vi "HFRR ADV v07 new software.vi"() -> ()   [LabVIEW 2025] (continued)
                    n2724 = Concatenate Strings(w3585, ".xls" ("string")) -> (w3583:string)
                  }
                  frame "csv" {
                    n2725 = Concatenate Strings(w3587, ".csv" ("string")) -> (w3588:string)
                  }
                  frame "txt" {
                    n2726 = Concatenate Strings(w3589, ".txt" ("string")) -> (w3590:string)
                  }
                }
                n2727 = local read "Test Date"() -> (w3581:string)
                n2728 = local read "String 45"() -> (w3495:string)
                n2729 = local read "String 31"() -> (w3580:string)
                n2730 = local read "String 32"() -> (w3579:string)
                n2731 = local read "TITTLE"() -> (w3503:string)
                n2732 = Number To Fractional String(number=w3550, width (-)=i16 6, precision (6)=i16 2) -> (F-format string=w3549:string)  [unwired: 1 in]
                n2733 = Number To Fractional String(number=w3564, width (-)=i16 6, precision (6)=i16 2) -> (F-format string=w3570:string)  [unwired: 1 in]
                n2734 = Number To Fractional String(number=w3565, width (-)=i16 6, precision (6)=i16 2) -> (F-format string=w3563:string)  [unwired: 1 in]
                n2735 = Number To Fractional String(number=w3569, width (-)=i16 6, precision (6)=i16 2) -> (F-format string=w3568:string)  [unwired: 1 in]
                n2736 = Number To Fractional String(number=w3561, width (-)=i16 6, precision (6)=i16 2) -> (F-format string=w3559:string)  [unwired: 1 in]
                n2737 = Number To Fractional String(number=w3562, width (-)=i16 6, precision (6)=i16 2) -> (F-format string=w3560:string)  [unwired: 1 in]
                n2738 = Number To Fractional String(number=w3573, width (-)=i16 6, precision (6)=i16 2) -> (F-format string=w3574:string)  [unwired: 1 in]
                n2739 = Number To Fractional String(number=w3577, precision (6)=i16 2) -> (F-format string=w3578:string)  [unwired: 2 in]
                n2740 = local read "s.NO"() -> (w3497:string)
                n2741 = Concatenate Strings("=" ("string"), w3503) -> (w3502:string)
                n2742 = Concatenate Strings("S.No," ("string"), "                                       Parameters" ("string")) -> (w3508:string)
                n2743 = Concatenate Strings(w3575, w3534, w3549, w3575, w3531, w3570, w3575, w3530, w3563, w3575, w3526, w3568, w3575, w3524, w3559, w3575, w3521, w3560, w3575, w3518, w3574, w3575, w3515, w3578) -> (w3537:string)
                n2744 = Concatenate Strings(w3507, "," ("string"), w3495, w3497, w3496, w3579, w3582, w3496, w3580, w3581, w3507) -> (w3505:string)
                n2745 = local read "Tested by"() -> (w3511:string)
                n2746 = local read "String 33"() -> (w3512:string)
                n2747 = Concatenate Strings("," ("string"), "                                                                             " ("string")) -> (w3500:string)
                n2748 = Concatenate Strings(w3502, w3498, w3505, w3498, w3508, w3537, w3498, w3500, w3512, w3511) -> (→"export":string)
                n2749 = String To Path(string=w3539) -> (path=w3546:path)
                n2750 = local read "export"() -> (w3541:string)
                n2751 = call <vilib>:"Write Characters To File.vi"("append to file? (new file:F)"=FALSE, "character string"=w3541, "file path (dialog if empty)"=w3546) -> ()  [unwired: 2 in, 1 out]
              }
            }
          }
          frame Enabled {
          }
        }
        n2752 = case shown="True" "OK Button 17" {
          frame False {
          }
          frame True {
            (unwired) 0  # existing file
            w3799 = "Choose a datalog file to open"  # prompt
            n2753 = local write "OK Button 17"(FALSE ("OK Button 17")) -> ()
            n2754 = local read "String"() -> (w3794:string)
            n2755 = String To Path(string=w3794) -> (path=w3795:path)
            n2756 = File Dialog(6:"*.duf" ("pattern"), 7:w3799, 11:w3795) -> (0:w3786:errorcluster, 3:w3805:path)  [unwired: 4 in, 2 out]
            n2757 = Unbundle(w3786) -> ()  [unwired: 3 out]
            n2758 = Open/Create/Replace File "Open File"(file path (use dialog)=w3805) -> (refnum out=w3797:refnum<file>)  [unwired: 5 in, 2 out]
            n2759 = Strip Path(path=w3805) -> (name=w3803:string)  [unwired: 1 out]
            n2760 = Path To String(path=w3805) -> (string=w3788:string)
            n2761 = while {
              tunnel: w3797 -> [w3809]
              i -> [w3806]
              stop <- w3807 continue-if-true
              (unwired) TRUE ("line mode (F)")
              n2762 = Read from Text File "Read File"(file (use dialog)=w3809) -> (text=w3808:string)  [unwired: 3 in, 3 out]
              n2763 = local write "Numeric 16"(w3806) -> ()
              n2764 = String Length(string=w3808) -> (length=w3811:i32)
              n2765 = Greater?(x=w3811, y=1) -> (0:w3807:bool)
            }
            n2766 = local write "String 29"(w3788) -> ()
            n2767 = Search and Replace String(input string=w3788, search string=".duf", replace string=".dgf" ("replace string (\"\")")) -> (result string=→"String Indicator 4":string)  [unwired: 5 in, 3 out]
            n2768 = Match Pattern(string=w3803, regular expression=".dwm") -> (before substring=w3787:string)  [unwired: 1 in, 3 out]
            "String Indicator" <- w3787
            n2769 = Match Pattern(string=w3788, regular expression=".dwm" ("substring (\"\")")) -> (before substring=w3789:string)  [unwired: 1 in, 3 out]
            "String Indicator 3" <- w3789
            n2770 = local write "TITTLE 2"(w3787) -> ()
            n2771 = String To Path(string=w3789) -> (path=w3796:path)
            "path" <- w3796
            n2772 = call <vilib>:"Read Characters From File.vi"("file path (dialog if empty)"=w3796, "start of read offset (chars.:0)"=60 ("start of read offset (chars.: 0)")) -> ("character string"=→"String Indicator 2":string)  [unwired: 4 in, 3 out]
          }
        }
        n2773 = call <vilib>:"Query Available Printers.vi"() -> ("system configured printers"=w3488:string[])  [unwired: 9 in, 2 out]
        "System Configured Printers 2" <- w3488
        n2774 = local read "OK Button 16"() -> (w3485:bool)
        n2775 = case shown="True" "OK Button 16" {
          frame False {
          }
          frame True {
            n2776 = stacked-sequence {
              frame #0 {
                n2777 = local read "Numeric 16"() -> (w3813:i32)
                n2778 = local write "Numeric 10"(w3813) -> ()
              }
              frame #1 {
                n2779 = local read "S.NO"() -> (→"s.NO":string)
                n2780 = local read "String 29"() -> (w3817:string)
                n2781 = String To Path(string=w3817) -> (path=w3816:path)
                n2782 = Open/Create/Replace File "Open File"(file path (use dialog)=w3816) -> (refnum out=w3818:refnum<file>)  [unwired: 5 in, 2 out]
                n2783 = for {
                  N: 16 -> [_]
                  tunnel: w3818 -> [w3825]
                  i -> [w3821]
                  (unwired) TRUE ("line mode (F)")
                  n2784 = Read from Text File "Read File"(file (use dialog)=w3825) -> (text=w3819:string)  [unwired: 3 in, 3 out]
                  n2785 = Match Pattern(string=w3819, regular expression="(") -> (after substring=w3824:string)  [unwired: 1 in, 3 out]
                  n2786 = Match Pattern(string=w3824, regular expression=")") -> (before substring=w3820:string)  [unwired: 1 in, 3 out]
                  n2787 = case shown="1" w3821 {
                    tunnel: w3820 -> [w3826 w3827 _ _ w3828 w3829 w3830 w3832 w3834 w3836 w3838 w3840 w3842 w3844 _]
                    tunnel: w3819 -> [_ _ _ _ _ _ _ _ _ _ _ _ _ _ _]
                    frame 0 {
                      "TITTLE" <- w3826
                    }
                    frame 1 {
                      "Sample ID" <- w3827
                    }
                    frame 2 {
                    }
                    frame 3 {
                    }
                    frame 4 {
                      "Test Date" <- w3828
                    }
                    frame 5 {
                      "Tested by" <- w3829
                    }
                    frame 6 {
                      n2788 = Fract/Exp String To Number(string=w3830) -> (number=→"Humidity before test 2":dbl)  [unwired: 3 in, 1 out]
                    }
                    frame 7 {
                      n2789 = Fract/Exp String To Number(string=w3832) -> (number=→"Temperature before test 2":dbl)  [unwired: 3 in, 1 out]
                    }
                    frame 8 {
                      n2790 = Fract/Exp String To Number(string=w3834) -> (number=→"Humidity after test 2":dbl)  [unwired: 3 in, 1 out]
                    }
                    frame 9 {
                      n2791 = Fract/Exp String To Number(string=w3836) -> (number=→"Temperature after test 2":dbl)  [unwired: 3 in, 1 out]
                    }
                    frame 10 {
                      n2792 = Fract/Exp String To Number(string=w3838) -> (number=→"MWSD 2":dbl)  [unwired: 3 in, 1 out]
                    }
                    frame 11 {
                      n2793 = Fract/Exp String To Number(string=w3840) -> (number=→"AVP 2":dbl)  [unwired: 3 in, 1 out]
                    }
                    frame 12 {
                      n2794 = Fract/Exp String To Number(string=w3842) -> (number=→"HCF 2":dbl)  [unwired: 3 in, 1 out]
                    }
                    frame 13 {
                      n2795 = Fract/Exp String To Number(string=w3844) -> (number=→"WS1.4 2":dbl)  [unwired: 3 in, 1 out]
                    }
                    frame 14, Default {
                    }
                  }
                }
              }
              frame #2 {
              }
            }
            n2796 = local write "OK Button 16"(FALSE ("OK Button 13")) -> ()
          }
        }
        n2797 = Index Array(array=w3488, index="Select Printer 3") -> (element=w3490:string)
        "Selected Printer" <- w3490
        n2798 = case shown="True" w3485 {
          frame False {
          }
          frame True {
            n2799 = flat-sequence {
              frame #0 {
              }
              frame #1 {
                n2800 = Wait (ms)(milliseconds to wait=u32 100) -> ()  [unwired: 1 out]
              }
              frame #2 {
                n2801 = local write "OK Button 16"(FALSE ("Print 3")) -> ()
              }
            }
          }
        }
        n2802 = case shown="True" "Print" {
          tunnel: w3490 -> [_ w3782]
          frame False {
          }
          frame True {
            (unwired) i16 6 ("width (-)")
            (unwired) "TESTED BY : "
            (unwired) "TESTED DATE :"
            (unwired) "SAMPLE ID : "
            (unwired) "SAMPLE DESIGN : "
            w3740 = "\r"
            w3757 = "\r"
            # "add image"
            n2803 = local read "Sample ID"() -> (w3730:string)
            n2804 = local read "Tested by"() -> (w3733:string)
            n2805 = local read "String 34"() -> (w3720:string)
            n2806 = local read "String 45"() -> (w3700:string)
            n2807 = local read "String 35"() -> (w3715:string)
            n2808 = local read "String 37"() -> (w3713:string)
            n2809 = local read "String 32"() -> (w3735:string)
            n2810 = local read "String 36"() -> (w3710:string)
            n2811 = local read "String 31"() -> (w3734:string)
            n2812 = local read "Test Date"() -> (w3731:string)
            n2813 = local read "String 33"() -> (w3736:string)
            n2814 = local read "String 38"() -> (w3706:string)
            n2815 = local read "String 39"() -> (w3703:string)
            n2816 = local write "Print"(FALSE ("Print FF")) -> ()
            n2817 = local read "S 39"() -> (w3718:string)
            n2818 = local read "S 38"() -> (w3725:string)
            n2819 = local read "Temperature before test 2"() -> (w3756:dbl)
            n2820 = local read "Temperature after test 2"() -> (w3746:dbl)
            n2821 = local read "Humidity before test 2"() -> (w3771:dbl)
            n2822 = local read "Humidity after test 2"() -> (w3755:dbl)
            n2823 = local read "MWSD 2"() -> (w3760:dbl)
            n2824 = local read "WS1.4 2"() -> (w3738:dbl)
            n2825 = Concatenate Strings("2)" ("string"), w3720) -> (w3721:string)
            n2826 = Concatenate Strings("3)" ("string"), w3718) -> (w3719:string)
            n2827 = Concatenate Strings("1)" ("string"), w3725) -> (w3724:string)
            n2828 = Concatenate Strings("4)" ("string"), w3715) -> (w3716:string)
            n2829 = Concatenate Strings("5)" ("string"), w3713) -> (w3712:string)
            n2830 = Concatenate Strings("6)" ("string"), w3710) -> (w3709:string)
            n2831 = Concatenate Strings("7)" ("string"), w3706) -> (w3707:string)
            n2832 = Concatenate Strings("8)" ("string"), w3703) -> (w3704:string)
            n2833 = local read "HCF 2"() -> (w3742:dbl)
            n2834 = local read "AVP 2"() -> (w3759:dbl)
            n2835 = local read "s.NO"() -> (w3701:string)
            n2836 = call <vilib>:"New Report.vi"("report type"=enum16{"Standard Report", "HTML"}."Standard Report") -> ("report out"=w3780:refnum<class "NI_report.lvclass">, "error out"=w3779:errorcluster)  [unwired: 13 in]
            n2837 = local read "TITTLE"() -> (w3732:string)
            n2838 = Concatenate Strings(w3757, w3700, w3701, w3757, w3735, w3730, w3757, w3734, w3731, w3757, w3736, w3733, w3757) -> (w3750:string)
            "test by" <- w3750
            n2839 = Number To Fractional String(number=w3756, width (-)=i16 6, precision (6)=i16 2) -> (F-format string=w3745:string)  [unwired: 1 in]
            n2840 = Number To Fractional String(number=w3755, width (-)=i16 6, precision (6)=i16 2) -> (F-format string=w3758:string)  [unwired: 1 in]
            n2841 = Number To Fractional String(number=w3771, width (-)=i16 6, precision (6)=i16 2) -> (F-format string=w3776:string)  [unwired: 1 in]
            n2842 = Number To Fractional String(number=w3760, width (-)=i16 6, precision (6)=i16 2) -> (F-format string=w3762:string)  [unwired: 1 in]
            n2843 = Number To Fractional String(number=w3746, width (-)=i16 6, precision (6)=i16 2) -> (F-format string=w3747:string)  [unwired: 1 in]
            n2844 = Number To Fractional String(number=w3759, width (-)=i16 6, precision (6)=i16 2) -> (F-format string=w3761:string)  [unwired: 1 in]
            n2845 = Number To Fractional String(number=w3742, width (-)=i16 6, precision (6)=i16 2) -> (F-format string=w3741:string)  [unwired: 1 in]
            n2846 = Number To Fractional String(number=w3738, precision (6)=i16 2) -> (F-format string=w3737:string)  [unwired: 2 in]
            n2847 = call-dynamic "Set Report Header Text.vi"("report in"=w3780, "center header text"=w3732, "error in (no error)"=w3779) -> ("report out"=w3751:refnum<class "NI_report.lvclass">, "error out"=w3752:errorcluster)  [unwired: 11 in]
            n2848 = Concatenate Strings(w3740, w3724, w3776, w3740, w3721, w3745, w3740, w3719, w3758, w3740, w3716, w3747, w3740, w3712, w3762, w3740, w3709, w3761, w3740, w3707, w3741, w3740, w3704, w3737) -> (w3728:string)
            "export 2" <- w3728
            n2849 = call-poly <vilib>:"Append Report Text.vi"("report in"=w3751, "text"=w3750, "error in (no error)"=w3752) -> ("report out"=w3754:refnum<class "NI_report.lvclass">, "error out"=w3753:errorcluster)  [unwired: 9 in, 2 out]
            n2850 = local read "test by"() -> (w3727:string)
            n2851 = local read "TITTLE"() -> (w3729:string)
            n2852 = call-poly <vilib>:"Append Report Text.vi"("report in"=w3754, "error in (no error)"=w3753) -> ("report out"=w3775:refnum<class "NI_report.lvclass">, "error out"=w3773:errorcluster)  [unwired: 10 in, 2 out]
            n2853 = Concatenate Strings(w3729, w3728, w3727) -> (→"output":string)
            n2854 = call-poly <vilib>:"Append Report Text.vi"("report in"=w3775, "text"=w3728, "error in (no error)"=w3773) -> ("report out"=w3774:refnum<class "NI_report.lvclass">, "error out"=w3772:errorcluster)  [unwired: 9 in, 2 out]
            n2855 = call-dynamic "Print Report.vi"("report in"=w3774, "printer name (default)"=w3782, "error in (no error)"=w3772) -> ("report out"=w3784:refnum<class "NI_report.lvclass">, "error out"=w3785:errorcluster)  [unwired: 11 in]
            n2856 = call-dynamic "Dispose Report.vi"("report in"=w3784, "error in (no error)"=w3785) -> ()  [unwired: 13 in, 1 out]
          }
        }
        n2857 = case shown="True" "Print 2" {
          frame False {
          }
          frame True {
            n2858 = flat-sequence {
              frame #0 {
                n2859 = local read "s.NO"() -> (→"s.NO 2":string)
                n2860 = Wait (ms)(milliseconds to wait=u32 20) -> ()  [unwired: 1 out]
                n2861 = local read "Sample ID  3"() -> (→"Sample ID  6":string)
                n2862 = local read "Sample ID  4"() -> (→"Sample ID  7":string)
                n2863 = local read "Sample ID"() -> (→"Sample ID  2":string)
                n2864 = local read "Tested by"() -> (→"Tested by 2":string)
                n2865 = local read "Test Date"() -> (→"Test Date 2":string)
                n2866 = local read "Humidity after test 3"() -> (→"Humidity after test 4":dbl)
                n2867 = local read "Ref A Test Date :"() -> (→"TITTLE 4":string)
                n2868 = local read "Temperature before test 3"() -> (w3607:dbl)
                n2869 = local read "Temperature before test 3"() -> (→"Temperature after test 5":dbl)
                n2870 = local read "Temperature after test 3"() -> (→"Temperature after test 4":dbl)
                n2871 = local read "Humidity before test 3"() -> (→"Humidity before test 4":dbl)
                n2872 = local write "Temperature before test 3"(w3607) -> ()
                n2873 = local read "image data"() -> (w3598:T13)
                n2874 = String To Path(string="C:\\LAB-IQ\\im\\Temp_resized.jpg") -> (path=w3599:path)
                "path 2" <- w3599
                n2875 = call <vilib>:"Write JPEG File.vi"("image data"=w3598, "path to JPEG file"=w3599) -> ()  [unwired: 8 in, 2 out]
                "Ref A Test Date :" <- "Ref A Test Date :"
                "Ref B Test Date :" <- "Ref B Test Date :"
                "Ref B Scar Value :" <- "Ref B Scar Value :"
                "Ref A Scar Value :" <- "Ref A Scar Value :"
              }
              frame #1 {
                (unwired) HTML_Report_Image_Alignment."MIDDLE" ("alignment (default)")
                w3635 = u16 0 items=["portrait", "landscape"] ("orientation (portrait)")
                (unwired) HTML_Report_Image_Alignment."ABSMIDDLE" ("alignment (default)")
                (unwired) "TESTED BY : "
                (unwired) "TESTED DATE :"
                (unwired) "SAMPLE ID : "
                (unwired) "SAMPLE DESIGN : "
                w3668 = "\r"
                # "add image"
                n2876 = Wait (ms)(milliseconds to wait=u32 20) -> ()  [unwired: 1 out]
                n2877 = local read "Sample ID  2"() -> (w3661:string)
                n2878 = local read "Wear Scar X"() -> (w3633:dbl)
                "Length ( microns ) 2" <- w3633
                n2879 = local read "Wear Scar Y"() -> (w3632:dbl)
                "Wear Scar Y ( microns ) :" <- w3632
                n2880 = local read "Test Date 2"() -> (w3662:string)
                n2881 = local read "Tested by 2"() -> (w3663:string)
                n2882 = local read "String 46"() -> (w3659:string)
                n2883 = local read "String 48"() -> (w3665:string)
                n2884 = local read "String 47"() -> (w3664:string)
                n2885 = local read "String 49"() -> (w3666:string)
                n2886 = local read "String 10"() -> (w3619:string)
                n2887 = local read "s.NO 2"() -> (w3660:string)
                n2888 = Add(x=w3633, y=w3632) -> (x+y=w3631:dbl)
                n2889 = call <vilib>:"New Report.vi"("report type"=enum16{"Standard Report", "HTML"}."HTML") -> ("report out"=w3639:refnum<class "NI_report.lvclass">, "error out"=w3637:errorcluster)  [unwired: 13 in]
                n2890 = Concatenate Strings(w3668, w3659, w3660, w3668, w3665, w3661, w3668, w3664, w3662, w3668, w3666, w3663, w3668) -> (→"test by 2":string)
                n2891 = Concatenate Strings("C:\\LAB-IQ\\Data\\" ("string"), w3619, ".jpg" ("string")) -> ()  [unwired: 1 out]
                n2892 = Divide(x=w3631, y=2.0) -> (x/y=→"Mean Wear ( microns) :":dbl)
                n2893 = call-dynamic "Set Report Orientation.vi"("report in"=w3639, "orientation (portrait)"=w3635, "error in (no error)"=w3637) -> ("report out"=w3638:refnum<class "NI_report.lvclass">, "error out"=w3636:errorcluster)  [unwired: 11 in]
                n2894 = for {
                  N: 5 -> [_]
                  tunnel: w3638 -> [w3689]
                  tunnel: [w3688] -> w3617
                  tunnel: w3636 -> [w3687]
                  tunnel: [w3686] -> w3616
                  n2895 = call-dynamic "Set Report Tab Width.vi"("report in"=w3689, "error in (no error)"=w3687) -> ("report out"=w3688:refnum<class "NI_report.lvclass">, "error out"=w3686:errorcluster)  [unwired: 12 in]
                }
                n2896 = local read "TITTLE"() -> (w3634:string)
                n2897 = call-dynamic "Set Report Header Text.vi"("report in"=w3617, "center header text"=w3634, "error in (no error)"=w3616) -> ("report out"=w3655:refnum<class "NI_report.lvclass">, "error out"=w3654:errorcluster)  [unwired: 11 in]
                n2898 = for {
                  N: 1 -> [_]
                  tunnel: [w3693] -> w3641
                  tunnel: [w3692] -> w3640
                  tunnel: w3655 -> [w3691]
                  tunnel: w3654 -> [w3690]
                  n2899 = call-dynamic "New Report Line.vi"("report in"=w3691, "error in (no error)"=w3690) -> ("report out"=w3693:refnum<class "NI_report.lvclass">, "error out"=w3692:errorcluster)  [unwired: 12 in]
                }
                n2900 = for {
                  N: 2 -> [_]
                  tunnel: [w3685] -> w3647
                  tunnel: [w3684] -> w3646
                  tunnel: w3641 -> [w3683]
                  tunnel: w3640 -> [w3682]
                  n2901 = call-dynamic "New Report Line.vi"("report in"=w3683, "error in (no error)"=w3682) -> ("report out"=w3685:refnum<class "NI_report.lvclass">, "error out"=w3684:errorcluster)  [unwired: 12 in]
                }
                n2902 = for {
                  N: 25 -> [_]
                  tunnel: w3647 -> [w3681]
                  tunnel: w3646 -> [w3679]
                  tunnel: [w3680] -> w3650
                  tunnel: [w3678] -> w3649
                  n2903 = call-dynamic "Set Report Tab Width.vi"("report in"=w3681, "error in (no error)"=w3679) -> ("report out"=w3680:refnum<class "NI_report.lvclass">, "error out"=w3678:errorcluster)  [unwired: 12 in]
                }
                n2904 = control-ref of="Tab Control 9"() -> (w3645:refnum<vi>)
                n2905 = call-dynamic "Append Control Image to Report.vi"("report in"=w3650, "alignment (default)"=HTML_Report_Image_Alignment."ABSMIDDLE", "ctrl reference"=w3645, "error in (no error)"=w3649) -> ("report out"=w3644:refnum<class "NI_report.lvclass">, "error out"=w3643:errorcluster)  [unwired: 8 in, 2 out]
                n2906 = for {
                  N: 3 -> [_]
                  tunnel: [w3677] -> w3628
                  tunnel: [w3676] -> w3627
                  tunnel: w3644 -> [w3675]
                  tunnel: w3643 -> [w3674]
                  n2907 = call-dynamic "New Report Line.vi"("report in"=w3675, "error in (no error)"=w3674) -> ("report out"=w3677:refnum<class "NI_report.lvclass">, "error out"=w3676:errorcluster)  [unwired: 12 in]
                }
                n2908 = for {
                  N: 100 -> [_]
                  tunnel: w3628 -> [w3673]
                  tunnel: w3627 -> [w3671]
                  tunnel: [w3672] -> w3624
                  tunnel: [w3670] -> w3622
                  n2909 = call-dynamic "Set Report Tab Width.vi"("report in"=w3673, "error in (no error)"=w3671) -> ("report out"=w3672:refnum<class "NI_report.lvclass">, "error out"=w3670:errorcluster)  [unwired: 12 in]
                }
                n2910 = String To Path(string="C:\\LAB-IQ\\im\\Temp_resized.jpg") -> (path=w3614:path)
                n2911 = call-poly <vilib>:"Append Image to Report.vi"("report in"=w3624, "path or URL of image"=w3614, "error in (no error)"=w3622) -> ("report out"=w3623:refnum<class "NI_report.lvclass">, "error out"=w3621:errorcluster)  [unwired: 9 in, 2 out]
                n2912 = call-poly <vilib>:"Open HTML Report in Browser.vi"("report in"=w3623, "error in (no error)"=w3621) -> ("report out"=w3658:refnum<class "NI_report.lvclass">, "error out"=w3657:errorcluster)  [unwired: 11 in, 1 out]
                n2913 = call-dynamic "Dispose Report.vi"("report in"=w3658, "error in (no error)"=w3657) -> ()  [unwired: 13 in, 1 out]
              }
              frame #2 {
              }
              frame #3 {
                n2914 = disable-structure shown="Disabled" {
                  frame Disabled {
                    n2915 = local read "String 10"() -> (w3698:string)
                    n2916 = Concatenate Strings("C:\\LAB-IQ-NXT\\Data\\" ("string"), w3698, ".jpg" ("string")) -> (w3696:string)
                    n2917 = String To Path(string=w3696) -> (path=w3695:path)
                    n2918 = Delete(path (use dialog)=w3695) -> ()  [unwired: 4 in, 3 out]
                  }
                  frame Enabled {
                  }
                }
                n2919 = local write "Print 2"(FALSE ("Print")) -> ()
              }
            }
          }
        }
      }
    }
    n2920 = property on="SetTemp" class="DigNum (strict)"("Disabled"=w1641) -> ()  [unwired: 2 in, 2 out]
    n2921 = Multiply(x=w1631, y=w1633) -> (x*y=w1632:dbl)
    n2922 = local read "MWSD"() -> (w1630:dbl)
    n2923 = Add(x=w1632, y=w1630) -> (x+y=→"WS1.4":dbl)
    n2924 = Wait (ms)(milliseconds to wait=u32 50) -> ()  [unwired: 1 out]
    n2925 = Wait (ms)(milliseconds to wait=u32 50) -> ()  [unwired: 1 out]
    n2926 = local read "Quit"() -> (w1629:bool)
  }
  n2927 = VISA Close(VISA resource name=w52, error in (no error)=w51) -> (error out=w49:errorcluster)
  n2928 = call <vilib>:"Clear Errors.vi"("error in (no error)"=w49) -> ()  [unwired: 5 in, 2 out]
  n2929 = VISA Close(VISA resource name=w37, error in (no error)=w36) -> ()  [unwired: 1 out]
  n2930 = while {
    tunnel: [w3857] -> w46
    shift-right: [w3850] -> _
    shift-left: 0.0 -> [w3853]
    shift-right: [w3849] -> _
    shift-left: 0.0 -> [w3852]
    shift-right: [w3848] -> _
    shift-left: 400.0 ("vc_cmd") -> [w3851]
    stop <- w3857 stop-if-true
    # "PID LOGIC"
    n2931 = local read "RUN"() -> (w3855:bool)
    n2932 = local read "Auto Start Test"() -> (w3854:bool)
    n2933 = local read "START TEMP"() -> (w3846:bool)
    n2934 = Or(x=w3855, y=w3854) -> (x .or. y?=w3856:bool)
    n2935 = And(x=w3856, y=w3846) -> (x .and. y?=w3847:bool)
    n2936 = Wait (ms)(milliseconds to wait=u32 20) -> ()  [unwired: 1 out]
    n2937 = case shown="True" w3847 {
      tunnel: [400.0 ("out_vc_cmd") w3877] -> w3848
      tunnel: [w3860 w3879] -> w3849
      tunnel: [w3860 w3878] -> w3850
      tunnel: w3853 -> [_ w3868]
      tunnel: w3852 -> [_ w3867]
      tunnel: w3851 -> [_ w3866]
      frame False {
        w3860 = 0.0 ("error_out")
      }
      frame True {
        n2938 = local read "Set Strk"() -> (w3863:dbl)
        n2939 = local read "LVDT STROKE"() -> (w3861:dbl)
        n2940 = Add(x=w3863, y="Add up Stroke") -> (x+y=w3864:dbl)
        n2941 = formula code="// Zero-Hardcode Explicit Positional-Form PID Engine\n// Inputs: target_stroke, measured_stroke, dt, prev_error, integral_accumulator_in, prev_vc_cmd\n//         kp, ki, kd, max_step_change, max_amplitude, min_amplitude, startup_cmd\n// Outputs: vc_cmd, error_out, out_error, integral_accumulator_out, out_vc_cmd\n\n// 1. Calculate Tracking Error\nfloat current_error = target_stroke - measured_stroke;\nerror_out = current_error;\n\n// 2. Compute Proportional Term\nfloat p_term = kp * current_error;\n\n// 3. Compute Derivative Term\nfloat d_term = 0.0;\nif (dt > 0.0) {\n    d_term = kd * ((current_error - prev_error) / dt);\n}\n\n// 4. Update and Accumulate Integral Term\nfloat current_integral = integral_accumulator_in + (current_error * dt);\nfloat i_term = ki * current_integral;\n\n// 5. Calculate Ideal Target Command\nfloat ideal_command = startup_cmd + p_term + i_term + d_term;\n\n// 6. Anti-Windup Protection (Back-calculation method)\nif (ideal_command > max_amplitude) {\n    float excess = ideal_command - max_amplitude;\n    if (ki > 0.0) {\n        current_integral -= excess / ki;\n    }\n    ideal_command = max_amplitude;\n} else if (ideal_command < min_amplitude) {\n    float excess = ideal_command - min_amplitude;\n    if (ki > 0.0) {\n        current_integral -= excess / ki;\n    }\n    ideal_command = min_amplitude;\n}\n\n// 7. Apply Loop Rate Limiting (Protects voice coil from large voltage steps)\nfloat raw_adjustment = ideal_command - prev_vc_cmd;\n\nif (raw_adjustment > max_step_change) {\n    raw_adjustment = max_step_change;\n} else if (raw_adjustment < -max_step_change) {\n    raw_adjustment = -max_step_change;\n}\n\nfloat next_vc_cmd = prev_vc_cmd + raw_adjustment;\n\n// Final Output Safety Safeguard Clamping\nif (next_vc_cmd > max_amplitude) {\n    next_vc_cmd = max_amplitude;\n} else if (next_vc_cmd < min_amplitude) {\n    next_vc_cmd = min_amplitude;\n}\n\n// 8. Map to Shift Registers for memory persistence\nvc_cmd = next_vc_cmd;\nout_error = current_error;                     \nintegral_accumulator_out = current_integral;  \nout_vc_cmd = next_vc_cmd;"("target_stroke"=w3864, "measured_stroke"=w3861, "dt"="dt", "integral_accumulator_in"=w3867, "prev_error"=w3868, "prev_vc_cmd"=w3866, "kp"="kp", "ki"="ki", "kd"="kd", "max_step_change"="max_step_change", "max_amplitude"="max_amplitude", "min_amplitude"="min_amplitude", "startup_cmd"="startup_cmd") -> ("vc_cmd"=w3883:dbl, "out_error"=w3878:dbl, "integral_accumulator_out"=w3879:dbl, "out_vc_cmd"=w3877:dbl)  [unwired: 1 out]
        "output Vpp" <- w3883
        n2942 = Number To Fractional String(number=w3883, precision (6)=i16 1) -> (F-format string=w3881:string)  [unwired: 2 in]
        n2943 = Concatenate Strings("DAC;" ("string"), w3881) -> (w3865:string)
        n2944 = local write "Command"(w3865) -> ()
        "prev_error" <- w3868
        "integral_accumulator_in" <- w3867
        "prev_vc_cmd" <- w3866
      }
    }
    n2945 = local read "Quit"() -> (w3857:bool)
  }
  n2946 = Or(x=w42, y=w41) -> (x .or. y?=w43:bool)
  n2947 = Or(x=w39, y=w43) -> (x .or. y?=w48:bool)
  n2948 = control-ref of="new picture"() -> ()  [unwired: 1 out]
  n2949 = Or(x=w54, y=w48) -> (x .or. y?=w45:bool)
  n2950 = Or(x=w45, y=w46) -> (x .or. y?=w40:bool)
  n2951 = while {
    tunnel: [w3884] -> w53
    i -> [w3891]
    stop <- w3884 stop-if-true
    n2952 = local read "Quit"() -> (w3884:bool)
    n2953 = Equal To 0?(x=w3891) -> (x = 0?=w3889:bool)
    n2954 = call "Elapsed Time3"("Time Target (s)"=45.0, "Auto Reset"=TRUE) -> ("Time has Elapsed"=w3888:bool)  [unwired: 10 in, 7 out]
    n2955 = Wait (ms)(milliseconds to wait=u32 50) -> ()  [unwired: 1 out]
    n2956 = Or(x=w3888, y=w3889) -> (x .or. y?=w3890:bool)
    n2957 = case shown="True" w3890 {
      frame False {
      }
      frame True {
        n2958 = call <vilib>:"System Exec.vi"("run minimized? (F)"=TRUE, "error in (no error)"="error in (no error)", "command line"="powercfg.exe -change -monitor-timeout-ac 0") -> ("error out"=w3902:errorcluster)  [unwired: 5 in, 3 out]
        n2959 = call <vilib>:"System Exec.vi"("run minimized? (F)"=TRUE, "error in (no error)"=w3902, "command line"="powercfg.exe -change -disk-timeout-ac 0") -> ("error out"=w3901:errorcluster)  [unwired: 5 in, 3 out]
        n2960 = call <vilib>:"System Exec.vi"("run minimized? (F)"=TRUE, "error in (no error)"=w3901, "command line"="powercfg.exe -change -standby-timeout-ac 0") -> ("error out"=w3900:errorcluster)  [unwired: 5 in, 3 out]
        n2961 = call <vilib>:"System Exec.vi"("run minimized? (F)"=TRUE, "error in (no error)"=w3900, "command line"="powercfg.exe -change -hibernate-timeout-ac 0") -> ("error out"=w3899:errorcluster)  [unwired: 5 in, 3 out]
        n2962 = call <vilib>:"Simple Error Handler.vi"("error in (no error)"=w3899) -> ("error out"=w3905:errorcluster)  [unwired: 4 in, 4 out]
        n2963 = call <vilib>:"Clear Errors.vi"("error in (no error)"=w3905) -> ("error out"=→"error out":errorcluster)  [unwired: 5 in, 1 out]
      }
    }
  }
  n2964 = Compound Arithmetic op=OR(w56, w40, w53) -> (w55:bool)
  n2965 = flat-sequence {
    tunnel: w55 -> [_]
    tunnel: [w3907] -> w18
    tunnel: w18 -> [_]
    frame #0 {
      n2966 = call "CLOSE CONNECTION.vi"() -> ("error out"=w3907:errorcluster)  [unwired: 11 in]
    }
    frame #1 {
      n2967 = Quit LabVIEW(quit? (T)=TRUE) -> ()
      n2968 = local write "Quit"(FALSE ("EXIT")) -> ()
    }
  }
  n2969 = property on="Heater Button" class="Bool (strict)"("Visible"=TRUE) -> ()  [unwired: 2 in, 2 out]
  n2970 = disable-structure shown="Disabled" {
    disable-tunnel: _ -> [w3913 _]
    disable-tunnel: _ -> [w3910 _]
    disable-tunnel: _ -> [w3911 _]
    frame Disabled {
      n2971 = disable-structure shown="Disabled" {
        disable-tunnel: [w3920 _] -> w3912
        frame Disabled {
          n2972 = while {
            shift-right: [w3962] -> w3918
            shift-left: errorcluster {"status"=TRUE, "code"=0, "source"="Init"} ("error out") -> [w3927]
            shift-right: [w3961] -> w3917
            shift-left: _ -> [w3928]
            shift-right: [w3960] -> _
            shift-left: "" -> [w3959]
            tunnel: [w3921] -> w3920
            shift-right: ["Set Rh"] -> _
            shift-left: 0.0 ("Set Rh") -> [w3953]
            tunnel: [w3930] -> _
            i -> [w3930]
            stop <- w3921 stop-if-true
            n2973 = flat-sequence {
              tunnel: w3927 -> [w3965]
              tunnel: [w3965] -> w3926
              frame #0 {
                n2974 = Wait (ms)(milliseconds to wait=u32 200) -> ()  [unwired: 1 out]
              }
            }
            n2975 = local read "Com Port 3"() -> (w3929:refnum<visa-resource-name>)
            n2976 = local read "Humidity Str Rec"() -> (w3931:string)
            n2977 = Not Equal?(x="Set Rh", y=w3953) -> (x != y?=w3958:bool)
            n2978 = Number To Decimal String(number="Set Rh") -> (decimal integer string=w3956:string)  [unwired: 1 in]
            n2979 = Not Equal?(x=w3929, y=w3928) -> (x != y?=w3924:bool)
            n2980 = Concatenate Strings("#setPoint00" ("string"), w3956) -> (w3957:string)
            n2981 = case shown="False" w3958 {
              tunnel: w3957 -> [_ w3977]
              frame False {
                n2982 = local read "Humidity"() -> (w3974:bool)
                n2983 = case shown="True" w3974 {
                  frame False {
                    n2984 = local write "Humidity Str Send"("stop" ("Humidity Str Send")) -> ()
                  }
                  frame True {
                    n2985 = local write "Humidity Str Send"("start" ("Humidity Str Send")) -> ()
                  }
                }
              }
              frame True {
                n2986 = local write "Humidity Str Send"(w3977) -> ()
              }
            }
            n2987 = Or(x=w3924) -> (y=w3922:bool, x .or. y?=w3923:bool)
            n2988 = String Subset(string=w3931, offset (0)=7) -> (substring=w3946:string)  [unwired: 1 in]
            n2989 = Match Pattern(string=w3931, regular expression="?") -> (offset past match=w3949:i32)  [unwired: 1 in, 3 out]
            n2990 = Match Pattern(string=w3931, regular expression="v") -> (offset past match=w3952:i32)  [unwired: 1 in, 3 out]
            n2991 = case shown="True" w3923 {
              tunnel: w3926 -> [w3963 _]
              tunnel: [w3963 errorcluster {"status"=TRUE, "code"=0, "source"="Init"} ("error out")] -> w3925
              frame False {
              }
              frame True {
              }
            }
            n2992 = Equal?(x=w3949, y=-1) -> (x = y?=w3933:bool)
            n2993 = Match Pattern(string=w3946, regular expression="g") -> (after substring=w3947:string, offset past match=w3938:i32)  [unwired: 1 in, 2 out]
            n2994 = Match Pattern(string=w3946, regular expression="y") -> (after substring=w3945:string, offset past match=w3939:i32)  [unwired: 1 in, 2 out]
            n2995 = Greater?(x=w3939, y=w3938) -> (0:w3944:bool)
            n2996 = Greater Or Equal To 0?(x=w3939) -> (x >= 0?=w3936:bool)
            n2997 = Greater Or Equal To 0?(x=w3938) -> (x >= 0?=w3937:bool)
            n2998 = Or(x=w3936, y=w3937) -> (x .or. y?=w3935:bool)
            n2999 = Greater Or Equal To 0?(x=w3952) -> (x >= 0?=w3934:bool)
            n3000 = Select(t=w3945, s=w3944, f=w3947) -> (s? t:f=w3940:string)
            n3001 = case shown="Error" w3925 {
              selector: w3925 -> [w3990 w4036]
              tunnel: [w3988 w4029] -> w3962
              tunnel: w3928 -> [w3991 w4035]
              tunnel: [w3989 w4038] -> w3961
              tunnel: w3959 -> [w3978 w4037]
              tunnel: [w3985 w4037] -> w3960
              frame No Error {
                n3002 = call "Elapsed Time7"() -> ("Time has Elapsed"=w3984:bool)  [unwired: 12 in, 7 out]
                n3003 = Not Equal?(x="Humidity Str Send", y=w3978) -> (x != y?=w3980:bool)
                n3004 = Or(x=w3980, y=w3984) -> (x .or. y?=w3983:bool)
                n3005 = Select(t="Humidity Str Send", s=w3980, f="vals" ("regular expression")) -> (s? t:f=w3979:string)
                n3006 = Or(x=w3983, y="Send") -> (x .or. y?=w3987:bool)
                n3007 = case shown="True" w3987 {
                  tunnel: [w3994 w3999] -> w3988
                  tunnel: w3991 -> [w3993 w4007]
                  tunnel: w3990 -> [w3994 w4006]
                  tunnel: [w3993 w4000] -> w3989
                  tunnel: w3979 -> [_ w4005]
                  tunnel: [w3992 w3996] -> w3985
                  tunnel: "Humidity Str Send" -> [_ w3997]
                  tunnel: w3980 -> [_ w3998]
                  tunnel: w3978 -> [w3992 w3995]
                  frame False {
                  }
                  frame True {
                    n3008 = flat-sequence {
                      tunnel: w4007 -> [w4015]
                      tunnel: w4006 -> [w4014]
                      tunnel: w4005 -> [w4011]
                      tunnel: [w4013] -> w4004
                      tunnel: [w4012] -> w4003
                      tunnel: w4004 -> [w4018]
                      tunnel: w4003 -> [w4017]
                      tunnel: [w4018] -> w4002
                      tunnel: [w4017] -> w4001
                      tunnel: w4002 -> [w4025]
                      tunnel: w4001 -> [w4024]
                      tunnel: [w4023] -> w4000
                      tunnel: [w4022] -> w3999
                      frame #0 {
                        n3009 = local write "Ser Led"(TRUE ("Boolean 4")) -> ()
                        n3010 = Concatenate Strings(w4011, "\r") -> (w4010:string)
                        n3011 = VISA Write(VISA resource name=w4015, write buffer=w4010, error in (no error)=w4014) -> (VISA resource name out=w4013:refnum<visa-resource-name>, error out=w4012:errorcluster)  [unwired: 1 out]
                      }
                      frame #1 {
                        n3012 = Wait (ms)(milliseconds to wait="wait") -> ()  [unwired: 1 out]
                      }
                      frame #2 {
                        w4020 = FALSE ("Send")
                        n3013 = property class="Instr"(reference=w4025, error in=w4024) -> (reference out=w4026:refnum<visa-resource-name>, error out=w4027:errorcluster, "Serial Settings:Number of Bytes at Serial Port"=w4019:u32)
                        n3014 = local write "Send"(w4020) -> ()
                        n3015 = local write "Ser Led"(w4020) -> ()
                        n3016 = VISA Read(VISA resource name=w4026, byte count=w4019, error in (no error)=w4027) -> (VISA resource name out=w4023:refnum<visa-resource-name>, read buffer=→"Humidity Str Rec":string, error out=w4022:errorcluster)  [unwired: 1 out]
                      }
                    }
                    n3017 = Select(t=w3997, s=w3998, f=w3995) -> (s? t:f=w3996:string)
                  }
                }
              }
              frame Error {
                w4043 = u16 0 items=["None"=0, "XON/XOFF"=1, "RTS/CTS"=2, "DTR/DSR"=4] ("flow control")
                w4039 = u16 0 items=["None", "Odd", "Even", "Mark", "Space"] ("parity")
                w4042 = u16 10 items=["1.0"=10, "1.5"=15, "2.0"=20] ("stop bits")
                n3018 = VISA Close(VISA resource name=w4035, error in (no error)=w4036) -> (error out=w4034:errorcluster)
                n3019 = local write "humid"("" ("humid")) -> ()
                n3020 = local write "Humidity Str Rec"("" ("Humidity Str Rec")) -> ()
                n3021 = call <vilib>:"Clear Errors.vi"("error in (no error)"=w4034) -> ("error out"=w4033:errorcluster)  [unwired: 5 in, 1 out]
                n3022 = local read "Com Port 3"() -> (w4032:refnum<visa-resource-name>)
                n3023 = call-poly "VISA Configure Serial Port"("VISA resource name"=w4032, "timeout (10sec)"=u32 1000, "termination char\n(0xA = '\\n' = LF)"=u8 10 ("termination char\n(0xA = '\\n' = LF)"), "Enable Termination\nChar (T)"=FALSE ("Enable Termination Char (T)"), "data bits (8)"=u16 8 ("data bits"), "parity (0:none)"=w4039, "error in (no error)"=w4033, "stop bits (10: 1 bit)"=w4042, "flow control (0:none)"=w4043) -> ("VISA resource name out"=w4038:refnum<visa-resource-name>, "baud rate (9600)"=w4030:u32, "error out"=w4029:errorcluster)  [unwired: 4 in]
              }
            }
            n3024 = Compound Arithmetic op=AND(w3934, w3933, w3935) -> (w3932:bool)
            n3025 = case shown="True" w3932 {
              tunnel: w3931 -> [_ _]
              tunnel: w3940 -> [_ w3970]
              frame False {
              }
              frame True {
                w3968 = " " ("regular expression")
                n3026 = Match Pattern(string=w3970, regular expression=" ") -> (after substring=w3972:string)  [unwired: 1 in, 3 out]
                n3027 = Match Pattern(string=w3972, regular expression=w3968) -> (before substring=→"humid":string, after substring=w3969:string)  [unwired: 1 in, 2 out]
                n3028 = Match Pattern(string=w3969, regular expression=w3968) -> (before substring=→"temp_@Rh sensor":string)  [unwired: 1 in, 3 out]
              }
            }
            n3029 = local read "Quit"() -> (w3921:bool)
          }
          n3030 = VISA Close(VISA resource name=w3917, error in (no error)=w3918) -> (error out=w3914:errorcluster)
          n3031 = call <vilib>:"Clear Errors.vi"("error in (no error)"=w3914) -> ()  [unwired: 5 in, 2 out]
        }
        frame Enabled {
        }
      }
    }
    frame Enabled {
    }
  }
  n3032 = while {
    tunnel: [w4050] -> _
    i -> [w4050]
    stop <- w4046 stop-if-true
    # "Langauage selection"
    n3033 = Equal?(x="Lan flag", y=22.0) -> ()  [unwired: 1 out]
    n3034 = disable-structure shown="Disabled" {
      frame Disabled {
        n3035 = stacked-sequence {
          frame #0 {
            n3036 = case shown="\"Russian\"" "Language Selection" {
              tunnel: [0 1] -> w4052
              frame "English", Default {
              }
              frame "Russian" {
              }
            }
            n3037 = for {
              N: 130 -> [_]
              tunnel: "Table" -> [w4061]
              tunnel: w4052 -> [w4060]
              i -> [w4059]
              n3038 = Index Array(array=w4061, index (row)=w4059, index (col)=w4060) -> (element=w4058:string)
              n3039 = case shown="123" w4059 {
                tunnel: w4058 -> [w4062 w4063 _ w4064 w4065 w4066 w4067 w4068 w4069 w4070 w4071 w4072 w4073 w4074 w4075 w4076 w4077 w4078 w4079 w4080 w4081 w4082 w4083 w4084 w4085 w4086 w4087 w4088 w4089 _ _ w4090 w4091 w4092 w4093 w4094 w4095 w4104 w4111 w4118 w4125 w4129 w4132 w4135 w4137 w4139 w4140 w4141 w4142 w4143 w4144 w4145 w4146 w4147 w4148 w4149 w4150 w4151 w4152 w4153 w4154 w4155 w4156 w4157 w4158 w4159 w4160 w4161 w4162 w4163 w4164 w4165 w4166 w4167 w4168 w4169 w4170 w4171 w4172 w4173 w4174 w4175 w4176 w4177 w4178 w4179 w4180 w4181 w4182 w4183 w4184 w4185 w4186 w4187 w4188 w4189 w4190 w4191 w4192 w4193 w4194 w4195 w4196 w4197 w4198 _ w4199 w4200 w4201 w4202 w4203 w4204 w4205 w4206 w4207 w4208 w4209 w4210 w4211 _ w4212 w4213 w4214 w4215 w4216 w4217 _]
                frame 0 {
                  n3040 = local write "S"(w4062) -> ()
                }
                frame 1 {
                  n3041 = local write "S 2"(w4063) -> ()
                }
                frame 2 {
                }
                frame 3 {
                  n3042 = local write "S 4"(w4064) -> ()
                }
                frame 4 {
                  n3043 = property on="FILE" class="Str"("Caption.Text"=w4065) -> ()  [unwired: 2 in, 2 out]
                }
                frame 5 {
                  n3044 = property on="Fuel Discription :" class="Str"("Caption.Text"=w4066) -> ()  [unwired: 2 in, 2 out]
                }
                frame 6 {
                  n3045 = property on="Remarks :" class="Str"("Caption.Text"=w4067) -> ()  [unwired: 2 in, 2 out]
                }
                frame 7 {
                  n3046 = property on="Save & Continue" class="Bool (strict)"("Boolean Text.Text"=w4068) -> ()  [unwired: 2 in, 2 out]
                }
                frame 8 {
                }
                frame 9 {
                  n3047 = property on="Set Hz" class="DigNum (strict)"("Caption.Text"=w4070) -> ()  [unwired: 2 in, 2 out]
                }
                frame 10 {
                  "String 3" <- w4071
                }
                frame 11 {
                  n3048 = property on="NORMAL LOAD" class="DigNum (strict)"("Caption.Text"=w4072) -> ()  [unwired: 2 in, 2 out]
                }
                frame 12 {
                  "String 5" <- w4073
                }
                frame 13 {
                  n3049 = property on="Set Temp" class="DigNum (strict)"("Caption.Text"=w4074) -> ()  [unwired: 2 in, 2 out]
                }
                frame 14 {
                  n3050 = local write "S 15"(w4075) -> ()
                }
                frame 15 {
                  n3051 = property on="Set Rh" class="DigNum (strict)"("Caption.Text"=w4076) -> ()  [unwired: 2 in, 2 out]
                }
                frame 16 {
                  "String 13" <- w4077
                  "String 26" <- w4077
                }
                frame 17 {
                  n3052 = local write "S 18"(w4078) -> ()
                }
                frame 18 {
                  "String 17" <- w4079
                }
                frame 19 {
                  n3053 = property on="test time" class="DigNum (strict)"("Caption.Text"=w4080) -> ()  [unwired: 2 in, 2 out]
                }
                frame 20 {
                  "String 18" <- w4081
                  "String 22" <- w4081
                }
                frame 21 {
                  n3054 = property on="Elapsed time" class="DigNum (strict)"("Caption.Text"=w4082) -> ()  [unwired: 2 in, 2 out]
                }
                frame 22 {
                  n3055 = property on="Samplingtime 2" class="DigNum (strict)"("Caption.Text"=w4083) -> ()  [unwired: 2 in, 2 out]
                }
                frame 23 {
                  "String 21" <- w4084
                }
                frame 24 {
                  n3056 = property on="Countdown" class="DigNum (strict)"("Caption.Text"=w4085) -> ()  [unwired: 2 in, 2 out]
                }
                frame 25 {
                  n3057 = property on="Countdown 2" class="DigNum (strict)"("Caption.Text"=w4086) -> ()  [unwired: 2 in, 2 out]
                }
                frame 26 {
                  n3058 = property on="Engage" class="Bool (strict)"("Boolean Text.Text"=w4087) -> ()  [unwired: 2 in, 2 out]
                }
                frame 27 {
                  n3059 = property on="Boolean  4" class="Bool (strict)"("Boolean Text.Text"=w4088) -> ()  [unwired: 2 in, 2 out]
                }
                frame 28 {
                  n3060 = property on="Test \nStatus" class="Bool (strict)"("Boolean Text.Text"=w4089) -> ()  [unwired: 2 in, 2 out]
                }
                frame 29 {
                }
                frame 30 {
                }
                frame 31 {
                }
                frame 32 {
                  n3061 = property on="RSTCOF" class="Bool"("Boolean Text.Text"=w4091) -> ()  [unwired: 2 in, 2 out]
                  n3062 = property on="RST FF" class="Bool"("Boolean Text.Text"=w4091) -> ()  [unwired: 2 in, 2 out]
                  n3063 = property on="RST TEMP" class="Bool"("Boolean Text.Text"=w4091) -> ()  [unwired: 2 in, 2 out]
                  n3064 = property on="RSTV1 3" class="Bool"("Boolean Text.Text"=w4091) -> ()  [unwired: 2 in, 2 out]
                  n3065 = property on="rstv2" class="Bool"("Boolean Text.Text"=w4091) -> ()  [unwired: 2 in, 2 out]
                  n3066 = property on="RSTV1 2" class="Bool"("Boolean Text.Text"=w4091) -> ()  [unwired: 2 in, 2 out]
                  n3067 = property on="RST CP" class="Bool"("Boolean Text.Text"=w4091) -> ()  [unwired: 2 in, 2 out]
                }
                frame 33 {
                  "S 61" <- w4092
                }
                frame 34 {
                  "String 23" <- w4093
                }
                frame 35 {
                  n3068 = property on="Rh Before" class="DigNum (strict)"("Caption.Text"=w4094) -> ()  [unwired: 2 in, 2 out]
                }
                frame 36 {
                  n3069 = Match Pattern(string=w4095, regular expression=",") -> (before substring=→"bs":string, after substring=→"as":string)  [unwired: 1 in, 2 out]
                  n3070 = property on="Rh After" class="DigNum (strict)"("Caption.Text"=w4095) -> ()  [unwired: 2 in, 2 out]
                }
                frame 37 {
                  n3071 = Match Pattern(string=w4104, regular expression=",") -> (before substring=w4103:string, after substring=w4102:string)  [unwired: 1 in, 2 out]
                  "bs" <- w4103
                  "as" <- w4102
                  n3072 = Concatenate Strings(w4103, w4102) -> (w4099:string)
                  n3073 = property on="Humidity before test 2" class="DigNum (strict)"("Caption.Text"=w4099) -> ()  [unwired: 2 in, 2 out]
                  n3074 = property on="Humidity before test" class="DigNum (strict)"("Caption.Text"=w4099) -> ()  [unwired: 2 in, 2 out]
                  n3075 = Concatenate Strings(w4099, "=" ("string")) -> (w4100:string)
                  n3076 = local write "S 38"(w4100) -> ()
                }
                frame 38 {
                  n3077 = Match Pattern(string=w4111, regular expression=",") -> (before substring=w4110:string, after substring=w4109:string)  [unwired: 1 in, 2 out]
                  "bs" <- w4110
                  "as" <- w4109
                  n3078 = Concatenate Strings(w4110, w4109) -> (w4106:string)
                  n3079 = property on="Humidity after test 2" class="DigNum (strict)"("Caption.Text"=w4106) -> ()  [unwired: 2 in, 2 out]
                  n3080 = Concatenate Strings(w4106, "=" ("string")) -> (w4108:string)
                  n3081 = property on="Humidity after test" class="DigNum (strict)"("Caption.Text"=w4106) -> ()  [unwired: 2 in, 2 out]
                  n3082 = local write "S 39"(w4108) -> ()
                }
                frame 39 {
                  n3083 = Match Pattern(string=w4118, regular expression=",") -> (before substring=w4117:string, after substring=w4116:string)  [unwired: 1 in, 2 out]
                  "bs" <- w4117
                  "as" <- w4116
                  n3084 = Concatenate Strings(w4117, w4116) -> (w4113:string)
                  n3085 = property on="Temperature before test 2" class="DigNum (strict)"("Caption.Text"=w4113) -> ()  [unwired: 2 in, 2 out]
                  n3086 = property on="Temperature before test" class="DigNum (strict)"("Caption.Text"=w4113) -> ()  [unwired: 2 in, 2 out]
                  n3087 = Concatenate Strings(w4113, "=" ("string")) -> (→"String 34":string)
                }
                frame 40 {
                  n3088 = Match Pattern(string=w4125, regular expression=",") -> (before substring=w4124:string, after substring=w4123:string)  [unwired: 1 in, 2 out]
                  "bs" <- w4124
                  "as" <- w4123
                  n3089 = Concatenate Strings(w4124, w4123) -> (w4120:string)
                  n3090 = property on="Temperature after test 2" class="DigNum (strict)"("Caption.Text"=w4120) -> ()  [unwired: 2 in, 2 out]
                  n3091 = Concatenate Strings(w4120, "=" ("string")) -> (→"String 35":string)
                  n3092 = property on="Temperature after test" class="DigNum (strict)"("Caption.Text"=w4120) -> ()  [unwired: 2 in, 2 out]
                }
                frame 41 {
                  n3093 = property on="AVP" class="DigNum (strict)"("Caption.Text"=w4129) -> ()  [unwired: 2 in, 2 out]
                  n3094 = property on="AVP 2" class="DigNum (strict)"("Caption.Text"=w4129) -> ()  [unwired: 2 in, 2 out]
                  n3095 = Concatenate Strings(w4129, "=" ("string")) -> (→"String 36":string)
                }
                frame 42 {
                  n3096 = property on="MWSD" class="DigNum (strict)"("Caption.Text"=w4132) -> ()  [unwired: 2 in, 2 out]
                  n3097 = property on="MWSD 2" class="DigNum (strict)"("Caption.Text"=w4132) -> ()  [unwired: 2 in, 2 out]
                  n3098 = Concatenate Strings(w4132, "=" ("string")) -> (→"String 37":string)
                }
                frame 43 {
                  n3099 = property on="HCF 2" class="DigNum (strict)"("Caption.Text"=w4135) -> ()  [unwired: 2 in, 2 out]
                  n3100 = property on="HCF" class="DigNum (strict)"("Caption.Text"=w4135) -> ()  [unwired: 2 in, 2 out]
                  n3101 = Concatenate Strings(w4135, "=" ("string")) -> (→"String 38":string)
                }
                frame 44 {
                  n3102 = Concatenate Strings(w4137, "=" ("string")) -> (→"String 39":string)
                  n3103 = property on="WS1.4 2" class="DigNum (strict)"("Caption.Text"=w4137) -> ()  [unwired: 2 in, 2 out]
                  n3104 = property on="WS1.4" class="DigNum (strict)"("Caption.Text"=w4137) -> ()  [unwired: 2 in, 2 out]
                }
                frame 45 {
                  n3105 = property on="Save Results" class="Bool (strict)"("Boolean Text.Text"=w4139) -> ()  [unwired: 2 in, 2 out]
                }
                frame 46 {
                  n3106 = local write "S 47"(w4140) -> ()
                }
                frame 47 {
                  n3107 = local write "S 48"(w4141) -> ()
                }
                frame 48 {
                  n3108 = local write "S 49"(w4142) -> ()
                }
                frame 49 {
                  n3109 = local write "S 50"(w4143) -> ()
                }
                frame 50 {
                  n3110 = local write "S 51"(w4144) -> ()
                }
                frame 51 {
                  n3111 = local write "S 52"(w4145) -> ()
                }
                frame 52 {
                  n3112 = local write "S 53"(w4146) -> ()
                }
                frame 53 {
                  n3113 = local write "S 54"(w4147) -> ()
                }
                frame 54 {
                  n3114 = local write "S 55"(w4148) -> ()
                }
                frame 55 {
                  n3115 = local write "S 56"(w4149) -> ()
                }
